vi "SLT_DataProcess.vi"(8 "error in":errorcluster caption="错误输入（无错误）", 10 "Data in":T4[](array[typedef]), 11 "Cards":T2[](array[typedef])) -> (0 "error out":errorcluster caption="错误输出", 2 "采集实时值":T1)   [LabVIEW 2016]
uses:
  <vilib>/Analysis/NI_AALBase.lvlib
  <vilib>/Analysis/baseanly.llb/Mean (DBL).vi
  Ctrls/RealtimeValues.ctl
  <vilib>/Pansino Software/LabVIEW Architecture/Queue Management/PSARC_Queue Insert Element.vi
  Variables/SLT_GlobleVariables.vi
  Hardware Drivers/QX/DAQ_ReadBlock.ctl
  DAQ-Config/Controls/PSCHN_Channel Para.ctl
  DAQ-Config/Controls/PSCHN_Card Para.ctl
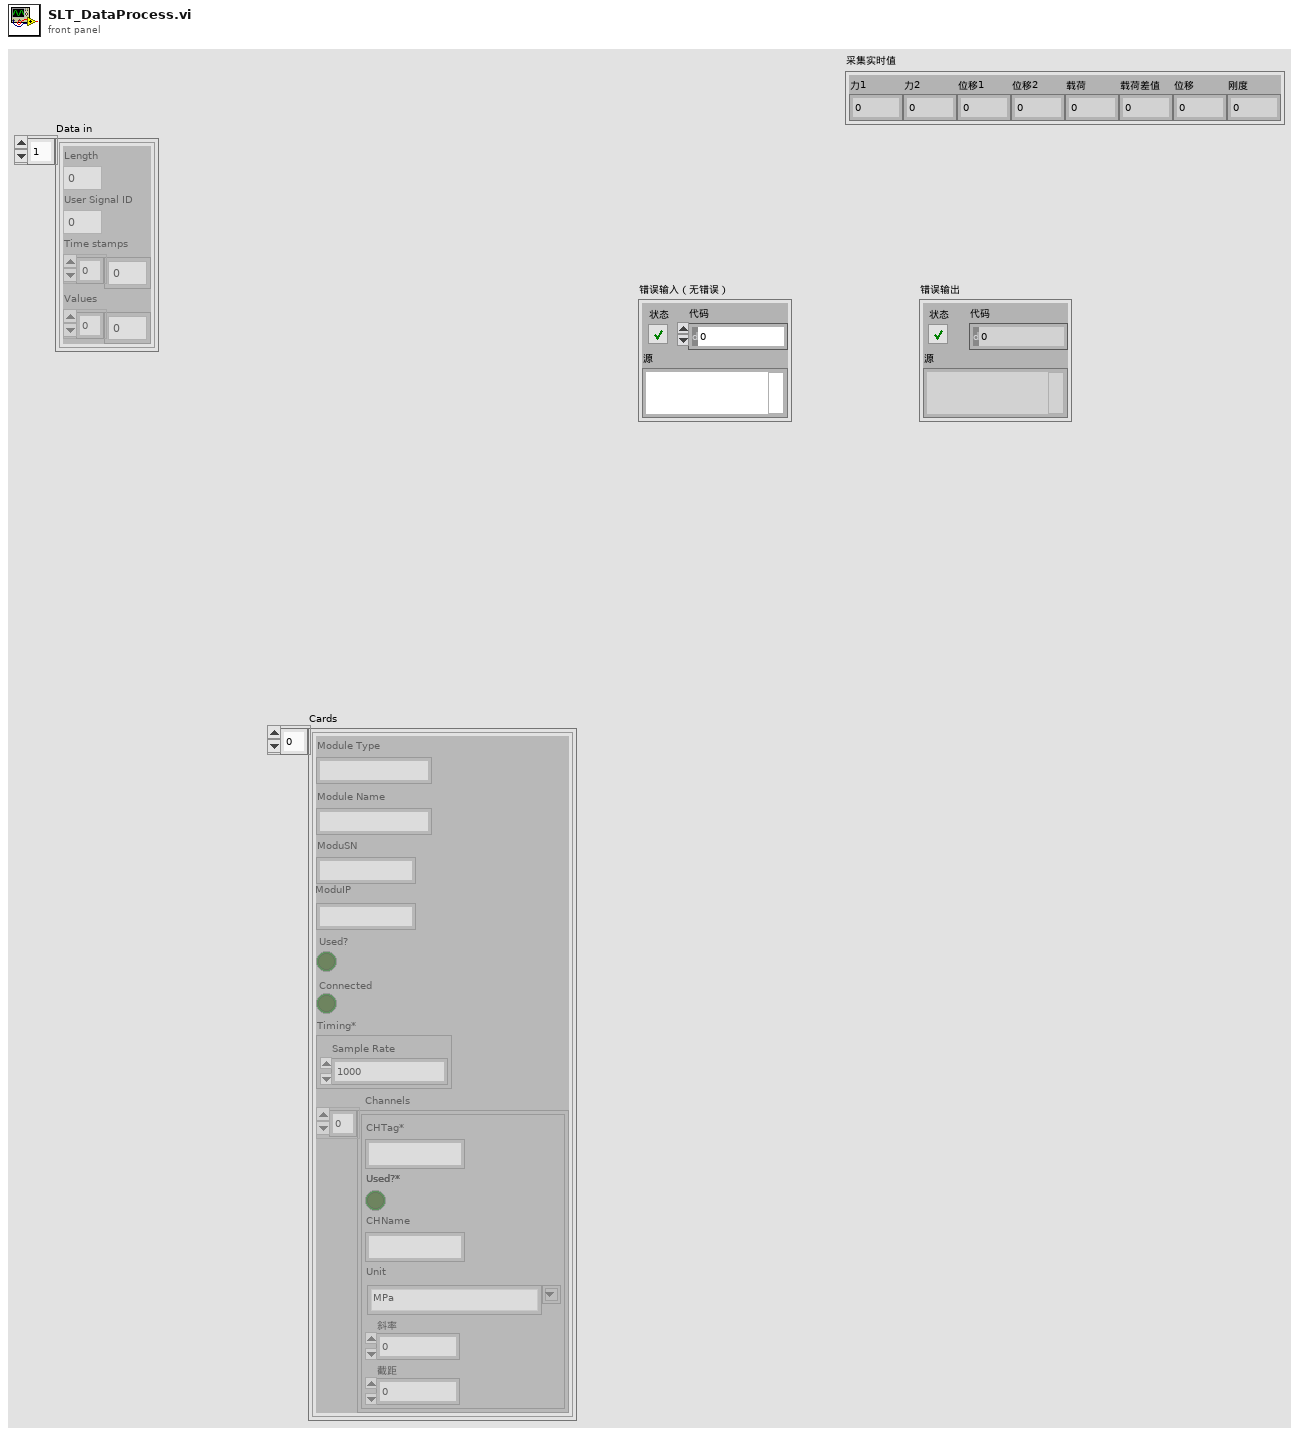
[diagram p1: front panel]
types:
  T1 = typedef "RealtimeValues.ctl" = cluster{"力1":dbl, "力2":dbl, "位移1":dbl, "位移2":dbl, "载荷":dbl, "载荷差值":dbl, "位移":dbl, "刚度":dbl}
  T2 = typedef "PSCHN_Card Para.ctl" = cluster{"Module Type":string, "Module Name":string, "ModuSN":string, "ModuIP":string, "Used?":bool, "Connected":bool, "Timing*":cluster{"Sample Rate":dbl}, "Channels":T3[]}
  T3 = typedef "PSCHN_Channel Para.ctl" = cluster{"CHTag*":string, "Used?*":bool, "CHName":string, "Unit":string, "斜率":dbl, "截距":dbl}
  T4 = typedef "DAQ_ReadBlock.ctl" = cluster{"Length":i32, "User Signal ID":i32, "Time stamps":dbl[], "Values":dbl[]}
  T5 = typedef "采集通道.ctl" = cluster{"力1通道":string, "力2通道":string, "位移1通道":string, "位移2通道":string}
  T6 = typedef "清零系数.ctl" = cluster{"力1清零系数":dbl, "力2清零系数":dbl, "位移1清零系数":dbl, "位移清零系数":dbl}
  T7 = cluster{"SLT Device Thread":string, "SLT Main Thread":string}
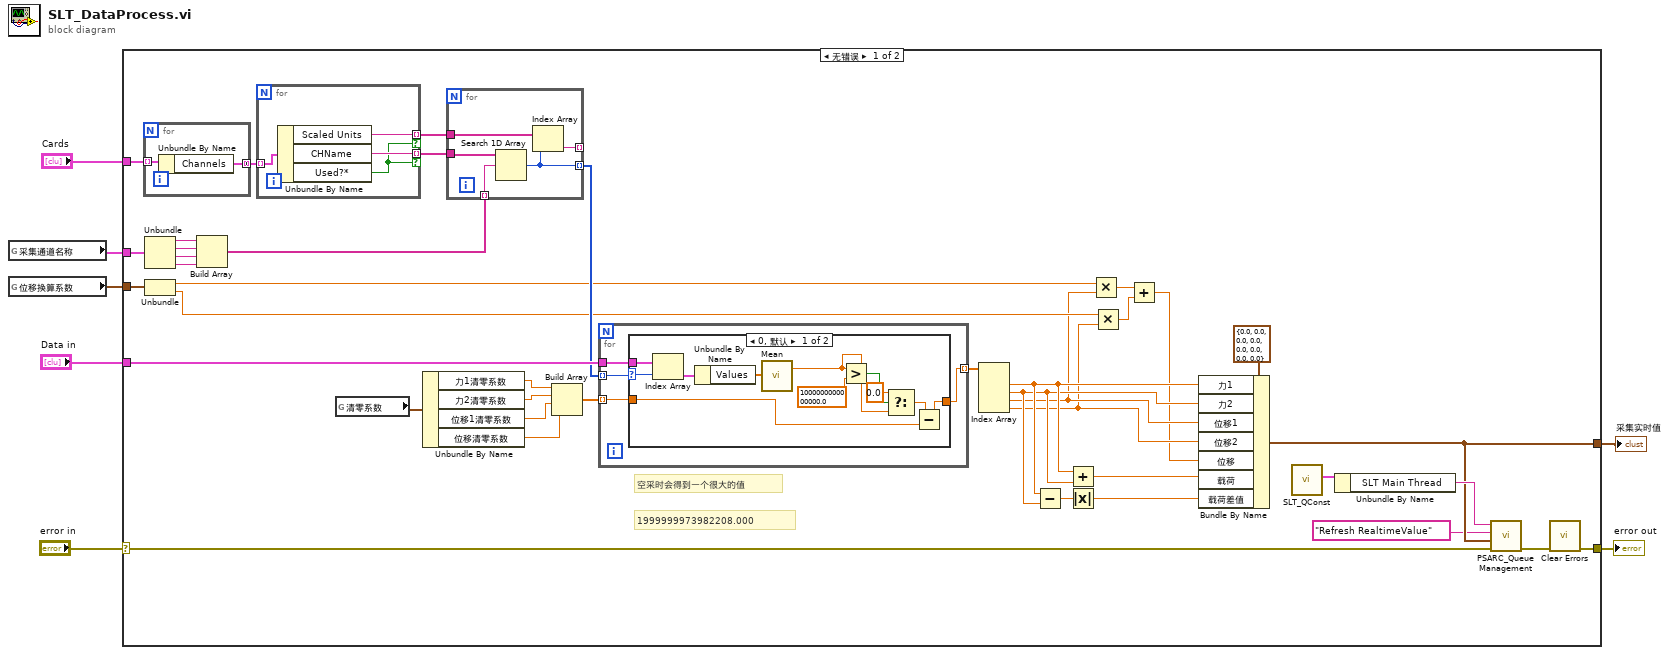
[diagram p0: block diagram]
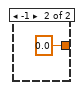
[diagram p2: hidden frame]
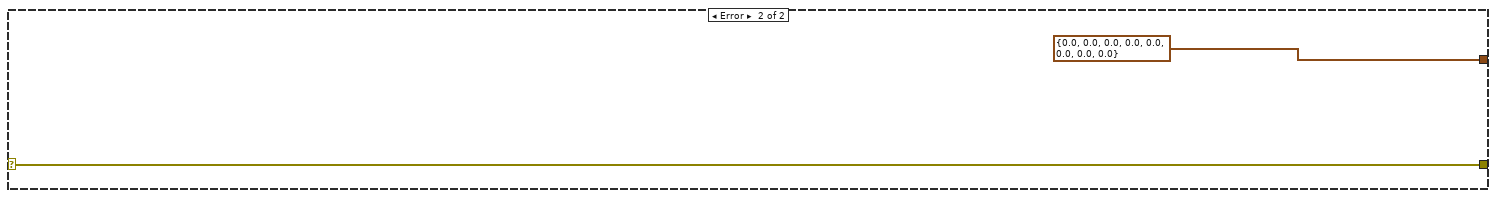
[diagram p3: hidden frame]
diagram:
  n1 = global read "SLT_GlobleVariables.vi" "采集通道名称"() -> (w2:T5)
  n2 = global read "SLT_GlobleVariables.vi" "位移换算系数"() -> (w1:cluster{"位移1系数":dbl, "位移2系数":dbl})
  n3 = case shown="无错误" "error in" {
    selector: "error in" -> [w25 w76]
    tunnel: [w22 w76] -> w6
    tunnel: "Data in" -> [w47 _]
    tunnel: "Cards" -> [w46 _]
    tunnel: w2 -> [w45 _]
    tunnel: [w26 T1 {"力1"=0.0, "力2"=0.0, "位移1"=0.0, "位移2"=0.0, "载荷"=0.0, "载荷差值"=0.0, "位移"=0.0, "刚度"=0.0} ("采集实时值")] -> w3
    tunnel: w1 -> [w21 _]
    frame No Error {
      # "空采时会得到一个很大的值"
      # "1999999973982208.000"
      n4 = for {
        tunnel: w46 -> [w49] mode=indexing
        tunnel: [w48] -> w39 mode=concatenating
        n5 = Unbundle By Name(w49) -> ("Channels"=w48:T3[])
      }
      n6 = Unbundle(w45) -> ("力1通道"=w44:string, "力2通道"=w43:string, "位移1通道"=w42:string, "位移2通道"=w41:string)
      n7 = Unbundle(w21) -> ("位移1系数"=w20:dbl, "位移2系数"=w19:dbl)
      n8 = Build Array(w44, w43, w42, w41) -> (w40:string[])
      n9 = for {
        tunnel: w39 -> [w58] mode=indexing
        tunnel: [w57] -> w37 mode=indexing if=w55
        tunnel: [w56] -> w38 mode=indexing if=w55
        n10 = Unbundle By Name(w58) -> ("Scaled Units"=w57:string, "CHName"=w56:string, "Used?*"=w55:bool)
      }
      n11 = global read "SLT_GlobleVariables.vi" "清零系数"() -> (w13:T6)
      n12 = Unbundle By Name(w13) -> ("力1清零系数"=w11:dbl, "力2清零系数"=w12:dbl, "位移1清零系数"=w10:dbl, "位移清零系数"=w9:dbl)
      n13 = for {
        tunnel: w38 -> [w54]
        tunnel: w37 -> [w53]
        tunnel: [w52] -> w36 mode=indexing
        tunnel: [w51] -> _ mode=indexing
        tunnel: w40 -> [w50] mode=indexing
        n14 = Search 1D Array(1D array=w54, element=w50) -> (index of element=w52:i32)  [unwired: 1 in]
        n15 = Index Array(array=w53, index=w52) -> (element=w51:string)
      }
      n16 = Build Array(w11, w12, w10, w9) -> (w8:dbl[])
      n17 = for {
        tunnel: w47 -> [w62]
        tunnel: w36 -> [w60] mode=indexing
        tunnel: [w61] -> w35 mode=indexing
        tunnel: w8 -> [w59] mode=indexing
        n18 = case shown="0, 默认" w60 {
          selector: w60 -> [w67 _]
          tunnel: w62 -> [w72 _]
          tunnel: [w64 0.0 ("mean")] -> w61
          tunnel: w59 -> [w63 _]
          frame 0, Default {
            n19 = Index Array(array=w72, index=w67) -> (element=w71:T4)
            n20 = Unbundle By Name(w71) -> ("Values"=w73:dbl[])
            n21 = call-poly <vilib>:"Mean.vi"("X"=w73) -> ("mean"=w66:dbl)  [unwired: 1 out]
            n22 = Greater?(x=w66, y=1000000000000000.0) -> (0:w69:bool)
            n23 = Select(t=0.0, s=w69, f=w66) -> (s? t:f=w65:dbl)
            n24 = Subtract(x=w65, y=w63) -> (x-y=w64:dbl)
          }
          frame -1 {
          }
        }
      }
      n25 = Index Array(array=w35) -> (element #1=w30:dbl, element #2=w29:dbl, element #3=w18:dbl, element #4=w17:dbl)  [unwired: 4 in]
      n26 = Subtract(x=w30, y=w29) -> (x-y=w32:dbl)
      n27 = Add(x=w30, y=w29) -> (x+y=w33:dbl)
      n28 = Absolute Value(x=w32) -> (abs(x)=w31:dbl)
      n29 = Multiply(x=w20, y=w18) -> (x*y=w16:dbl)
      n30 = Multiply(x=w19, y=w17) -> (x*y=w15:dbl)
      n31 = Add(x=w16, y=w15) -> (x+y=w14:dbl)
      n32 = Bundle By Name(cluster=T1 {"力1"=0.0, "力2"=0.0, "位移1"=0.0, "位移2"=0.0, "载荷"=0.0, "载荷差值"=0.0, "位移"=0.0, "刚度"=0.0} ("采集实时值"), "力1"=w30, "力2"=w29, "位移1"=w18, "位移2"=w17, "位移"=w14, "载荷"=w33, "载荷差值"=w31) -> (w26:T1)
      n33 = call "SLT_QConst.vi"() -> ("QNames"=w28:T7)  [unwired: 11 in]
      n34 = Unbundle By Name(w28) -> ("SLT Main Thread"=w27:string)
      n35 = call-poly <vilib>:"PSARC_Queue Management.vi"("error in (no error)"=w25, "Data"=w26, "Event"="Refresh RealtimeValue", "Queue Name(unamed)"=w27) -> ("error out"=w23:errorcluster)  [unwired: 6 in, 1 out]
      n36 = call <vilib>:"Clear Errors.vi"("error in (no error)"=w23) -> ("error out"=w22:errorcluster)  [unwired: 5 in, 1 out]
    }
    frame Error {
    }
  }
  "error out" <- w6
  "采集实时值" <- w3
